vi "createFromXml.vi"(8 "error in (no error)":errorcluster, 10 "dataPointXml":refnum<class "xmlNode.lvclass">) -> (0 "error out":errorcluster, 3 "ScriptEvent out":refnum<class "ScriptEvent.lvclass">)   [LabVIEW 2009, in "Tools.lvlib" / "Scripting.lvlib" / "ScriptEvent.lvclass"]
uses:
  ScriptEvent.lvclass
  xmlNode/xmlNode.lvclass
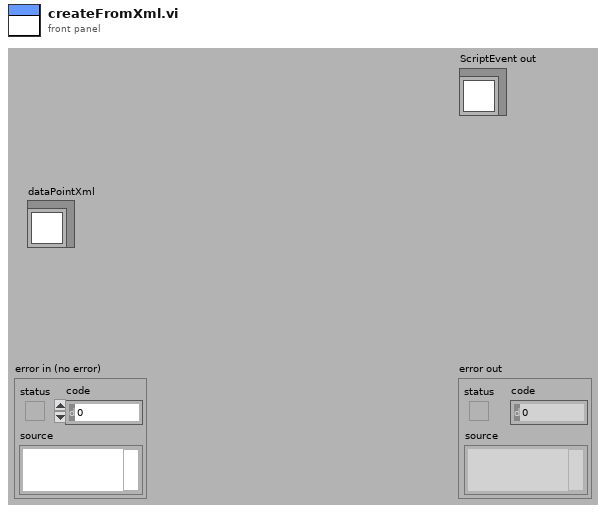
[diagram p1: front panel]
types:
  T1 = enum16{"changeValue", "pulse", "clock", "rampUp", "rampDown", "singleTone", "singleToneRamp", "playFile"}
  T2 = enum16{"changeValue", "pulse", "clock", "rampUp", "rampDown", "singleTone", "singleToneRamp", "playFile", "rf"}
  T3 = enum16{"changeValue", "pulse", "clock", "rampUp", "rampDown", "singleTone", "singleToneRamp", "playFile", "rf", "rfRamp"}
  T4 = enum16{"changeValue", "pulse", "clock", "rampUp", "rampDown", "singleTone", "singleToneRamp", "playFile", "rf", "rfRamp", "delay"}
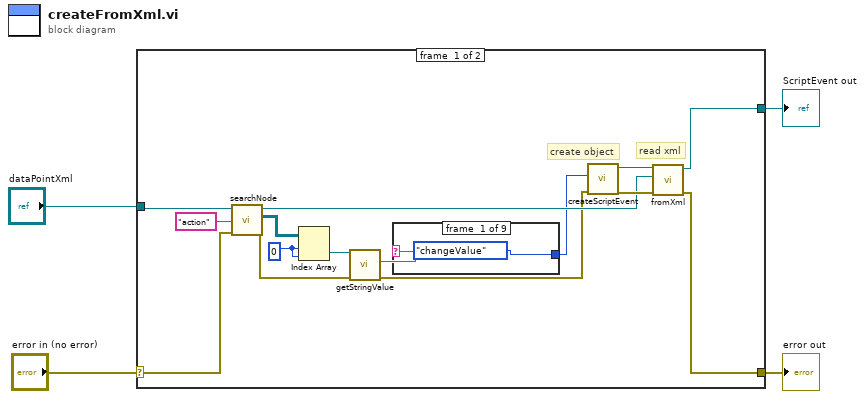
[diagram p0: block diagram]
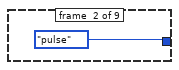
[diagram p2: hidden frame]
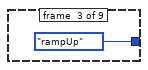
[diagram p3: hidden frame]
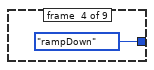
[diagram p4: hidden frame]
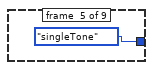
[diagram p5: hidden frame]
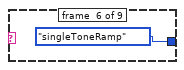
[diagram p6: hidden frame]
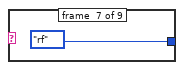
[diagram p7: hidden frame]
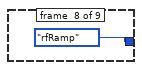
[diagram p8: hidden frame]
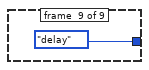
[diagram p9: hidden frame]
diagram:
  n1 = case shown="No Error" "error in (no error)" {
    selector: "error in (no error)" -> [w13 w29]
    tunnel: [w16 w29] -> w3
    tunnel: [w17 _] -> w2
    tunnel: "dataPointXml" -> [w15 _]
    frame #0 {
      w10 = 0
      # "read xml"
      # "create object"
      n2 = call-dynamic "searchNode.vi"("error in (no error)"=w13, "searchElementName"="action", "xmlNode in"=w15) -> ("error out"=w9:errorcluster, "arrayXmlNodes"=w12:refnum<class "xmlNode.lvclass">[][], "xmlNode out"=w7:refnum<class "xmlNode.lvclass">)  [unwired: 6 in]
      n3 = Index Array(array=w12, index (row)=w10, index (col)=w10) -> (element=w11:refnum<class "xmlNode.lvclass">)
      n4 = call-dynamic "getStringValue.vi"("error in (no error)"=w9, "xmlNode.lvclass in"=w11) -> ("error out"=w6:errorcluster, "stringValue"=w8:string)  [unwired: 7 in, 1 out]
      n5 = case shown="\"delay\"" w8 {
        tunnel: [T1."changeValue" ("action") T1."pulse" ("action") T1."rampUp" ("action") T1."rampDown" ("action") T1."singleTone" ("action") T1."singleToneRamp" ("action") T2."rf" ("action") T3."rfRamp" ("action") T4."delay" ("action")] -> w5
        frame #0 {
        }
        frame #1 {
        }
        frame #2 {
        }
        frame #3 {
        }
        frame #4 {
        }
        frame #5 {
        }
        frame #6 {
        }
        frame #7 {
        }
        frame #8 {
        }
      }
      n6 = call "createScriptEvent.vi"("error in (no error)"=w6, "action"=w5) -> ("error out"=w18:errorcluster, "ScriptEvent out"=w19:refnum<class "ScriptEvent.lvclass">)  [unwired: 8 in]
      n7 = call-dynamic "fromXml.vi"("error in (no error)"=w18, "dataPointXml"=w7, "ScriptEvent in"=w19) -> ("error out"=w16:errorcluster, "ScriptEvent out"=w17:refnum<class "ScriptEvent.lvclass">)  [unwired: 7 in]
    }
    frame #1 {
    }
  }
  "error out" <- w3
  "ScriptEvent out" <- w2
